vi "Helper Action.vi"(8 "error in (no error)":errorcluster, 9 "Message Data":variant, 10 "Message":string, 11 "Work Dispatcher In":refnum<class "Work Dispatcher.lvclass">) -> (0 "error out":errorcluster, 1 "Exit?":bool, 2 "Loop Period [ms]":u32=1000, 3 "Work Dispatcher Out":refnum<class "Work Dispatcher.lvclass">)   [LabVIEW 2020, in "Work Dispatcher.lvclass"]
doc: "The specific action implemented in the helper loop. Multiple different actions may be supported by using the Message and Message Data input to separate them. Any number of helper loops may run in parallell running the same or different actions. \nThe helper loop rate is controlled by the Loop Perid output of this method. \nIf this method throws an error, the helper loop will stop. The error will be sent to the error handler configured for the process. To stop it intentionally, the Stop Helper Loop.vi should be used. \nOne caveat with the helper loop is that it will have a copy of the object attributes as they were when the helper loop was started. If the attributes are updated, the helper loop will need to be restarted to refresh attributes."
uses:
  Work Dispatcher.lvclass
  Work Dispatcher.lvclass/Work Dispatcher.ctl
  People/Process Job/Job Handler.lvclass
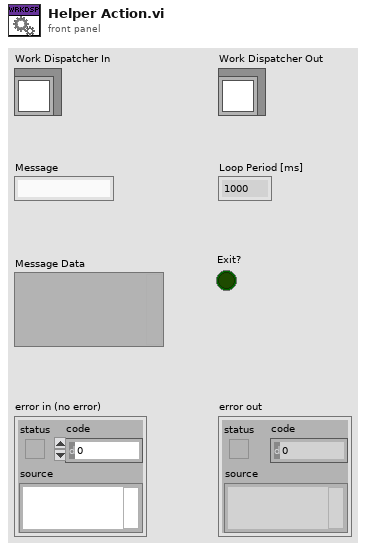
[diagram p1: front panel]
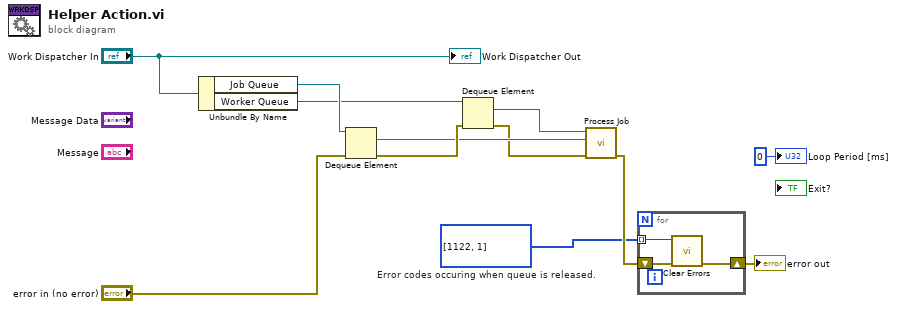
[diagram p0: block diagram]
diagram:
  w1 = i32[] [1122, 1]  # Error codes occuring when queue is released.
  n1 = Unbundle By Name("Work Dispatcher In") -> ("Job Queue"=w11:refnum<queue>, "Worker Queue"=w9:refnum<queue>)
  n2 = Dequeue Element(queue=w11, error in (no error)="error in (no error)") -> (element=w6:refnum<class>, error out=w8:errorcluster)  [unwired: 1 in, 2 out]
  n3 = Dequeue Element(queue=w9, error in (no error)=w8) -> (element=w7:refnum<class "Job Handler.lvclass">, error out=w5:errorcluster)  [unwired: 1 in, 2 out]
  n4 = call-dynamic "Process Job.vi"("error in (no error)"=w5, "Job"=w6, "Process Job In"=w7) -> ("error out"=w4:errorcluster)  [unwired: 7 in, 1 out]
  n5 = for {
    tunnel: w1 -> [w13] mode=indexing
    shift-right: [w14] -> w2
    shift-left: w4 -> [w15]
    n6 = call <vilib>:"Clear Errors.vi"("error in (no error)"=w15, "specific error code to clear (0: all)"=w13) -> ("error out"=w14:errorcluster)  [unwired: 4 in, 1 out]
  }
  "error out" <- w2
  "Work Dispatcher Out" <- "Work Dispatcher In"
  "Loop Period [ms]" <- u32 0 ("Loop Period [ms]")
